vi "Update State.vi"(7 "Process State":T1, 11 "CoolAppProcess in":refnum<class "CoolAppProcess.lvclass">) -> (3 "CoolAppProcess out":refnum<class "CoolAppProcess.lvclass">)   [LabVIEW 2020, in "LAF2024Q2.lvlib" / "CoolAppProcess.lvclass"]
uses:
  CoolAppProcess.lvclass
  C:/Program Files (x86)/National Instruments/LabVIEW 2020/vi.lib/ActorFramework/Actor/Actor.lvclass
  Process State.ctl
  CoolAppProcess.lvclass/CoolAppProcess.ctl
  <vilib>/ActorFramework/Actor/Actor.lvclass/Actor.ctl
  <vilib>/ActorFramework/Message Enqueuer/Message Enqueuer.lvclass/Message Enqueuer.ctl
  ProcStateHandler Messages/Handle State Msg/Handle State Msg.lvclass/Handle State Msg.ctl
  <vilib>/ActorFramework/Message Enqueuer/Init from Existing Queue.vi
  <vilib>/ActorFramework/Message Enqueuer/Enqueue.vi
  ProcStateHandler Messages/Handle State Msg/Handle State Msg.lvclass
  C:/Program Files (x86)/National Instruments/LabVIEW 2020/vi.lib/ActorFramework/Message/Message.lvclass
  <vilib>/ActorFramework/Message Priority Queue/Priority Enqueue.vi
  <vilib>/ActorFramework/Message Enqueuer/Message Enqueuer.lvclass
  <vilib>/ActorFramework/Actor/Actor.lvclass
  LAF2024Q2.lvlib
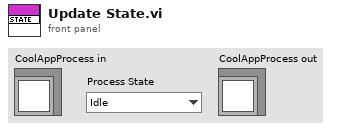
[diagram p1: front panel]
types:
  T1 = typedef "LAF2024Q2.lvlib/Process State.ctl" = enum16{"Idle", "Initializing", "Starting", "Running", "Stopping", "Stopped"}
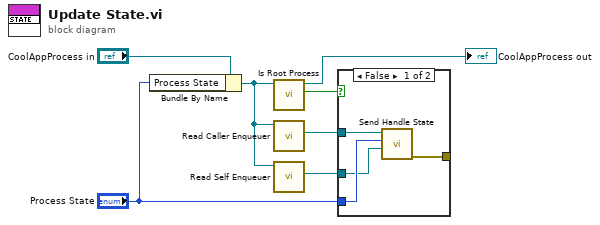
[diagram p0: block diagram]
diagram:
  n1 = Bundle By Name(cluster="CoolAppProcess in", "Process State"="Process State") -> (w2:refnum<class "CoolAppProcess.lvclass">)
  n2 = call "Is Root Process.vi"("CoolAppProcess in"=w2) -> ("Root Process"=w4:bool, "CoolAppProcess out"=→"CoolAppProcess out":refnum<class "CoolAppProcess.lvclass">)  [unwired: 8 in, 1 out]
  n3 = call <vilib>:"Read Caller Enqueuer.vi"("Actor"=w2) -> ("Caller Enqueuer"=w5:refnum<class "Message Enqueuer.lvclass">)  [unwired: 10 in]
  n4 = call <vilib>:"Read Self Enqueuer.vi"("Actor"=w2) -> ("Self Enqueuer"=w1:refnum<class "Message Enqueuer.lvclass">)  [unwired: 10 in]
  n5 = case shown="False" w4 {
    tunnel: w5 -> [w11 _]
    tunnel: "Process State" -> [w10 _]
    tunnel: w1 -> [w9 _]
    tunnel: [w8 _] -> _
    frame False {
      n6 = call "Send Handle State.vi"("Sender"=w9, "Process State"=w10, "Message Enqueuer"=w11) -> ("error out"=w8:errorcluster)  [unwired: 7 in, 1 out]
    }
    frame True {
    }
  }
